vi "rs3 capture single 2.vi"(0 "queue in":u64, 5 "timeout":u32=5000, 11 "error in (no error)":errorcluster) -> (1 "Capture Error":string="No Error", 2 "Frame number":u64, 3 "RS Format":u16(ring)=6 items=["    RS2_FORMAT_ANY             , /**< When passed to enable stream, librealsense will try to provide best suited format */", "    RS2_FORMAT_Z16             , /**< 16-bit linear depth values. The depth is meters is equal to depth scale * pixel value. */", "    RS2_FORMAT_DISPARITY16     , /**< 16-bit linear disparity values. The depth in meters is equal to depth scale / pixel value. */", "    RS2_FORMAT_XYZ32F          , /**< 32-bit floating point 3D coordinates. */", "    RS2_FORMAT_YUYV            , /**< Standard YUV pixel format as described in https://en.wikipedia.org/wiki/YUV */", "    RS2_FORMAT_RGB8            , /**< 8-bit red, green and blue channels */", "    RS2_FORMAT_BGR8            , /**< 8-bit blue, green, and red channels -- suitable for OpenCV */", "    RS2_FORMAT_RGBA8           , /**< 8-bit red, green and blue channels + constant alpha channel equal to FF */", "    RS2_FORMAT_BGRA8           , /**< 8-bit blue, green, and red channels + constant alpha channel equal to FF */", "    RS2_FORMAT_Y8              , /**< 8-bit per-pixel grayscale image */", "    RS2_FORMAT_Y16             , /**< 16-bit per-pixel grayscale image */", "    RS2_FORMAT_RAW10           , /**< Four 10-bit luminance values encoded into a 5-byte macropixel */", "    RS2_FORMAT_RAW16           , /**< 16-bit raw image */", "    RS2_FORMAT_RAW8            , /**< 8-bit raw image */", "    RS2_FORMAT_UYVY            , /**< Similar to the standard YUYV pixel format, but packed in a different order */", "    RS2_FORMAT_MOTION_RAW      , /**< Raw data from the motion sensor */", "    RS2_FORMAT_MOTION_XYZ32F   , /**< Motion data packed as 3 32-bit float values, for X, Y, and Z axis */", "    RS2_FORMAT_GPIO_RAW        , /**< Raw data from the external sensors hooked to one of the GPIO's */", "    RS2_FORMAT_COUNT             /**< Number of enumeration values. Not a valid input: intended to be used in for-loops. */"], 4 "RS Stream":u16(ring) items=["    RS2_STREAM_ANY,", "    RS2_STREAM_DEPTH                            , /**< Native stream of depth data produced by RealSense device */", "    RS2_STREAM_COLOR                            , /**< Native stream of color data captured by RealSense device */", "    RS2_STREAM_INFRARED                         , /**< Native stream of infrared data captured by RealSense device */", "    RS2_STREAM_FISHEYE                          , /**< Native stream of fish-eye (wide) data captured from the dedicate motion camera */", "    RS2_STREAM_GYRO                             , /**< Native stream of gyroscope motion data produced by RealSense device */", "    RS2_STREAM_ACCEL                            , /**< Native stream of accelerometer motion data produced by RealSense device */", "    RS2_STREAM_GPIO                             , /**< Signals from external device connected through GPIO */", "    RS2_STREAM_COUNT"], 6 "frame out":u64, 8 "width":i32, 9 "Blocking time, ms":u32, 10 "Stream type":T1(ring), 12 "index":i32, 13 "Time stamp":dbl, 14 "height":i32, 15 "error out":errorcluster)   [LabVIEW 2018, in "libRealSense3.lvlib"]
doc: "This VI waits for and returns the FRAME handle of captured data. (This is a BLOCKING call)\nIt also queries the frame profile to identify the type of stream data it was. \nThis type is output into the \"Stream Type\":\n\n0 Depth\n3 Color left\n5 IR Left \n9 IR Right\n21 IR Left (Y16)\n25 IR RIght (Y16)"
uses:
  libRealSense3.lvlib
panel:
  # "RS3 Capture Single 2"
  # "(C) Intel Corp. 2017,  AGJ"
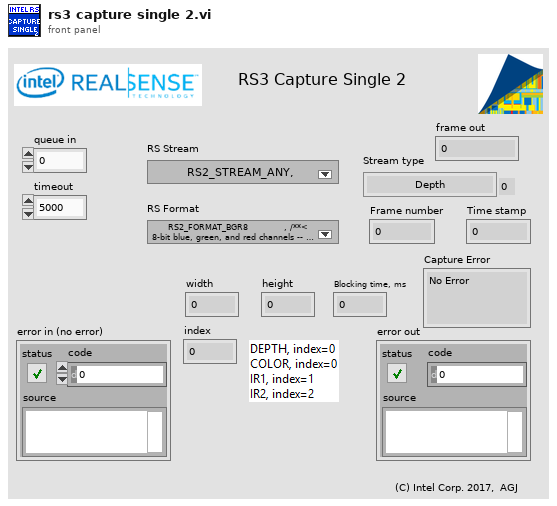
[diagram p1: front panel]
types:
  T1 = enum16{"Depth", "Color (ext.)", "Color (left) ", "IR Left", "IR Right", "IR Left (Y16)", "IR Right (Y16)"}
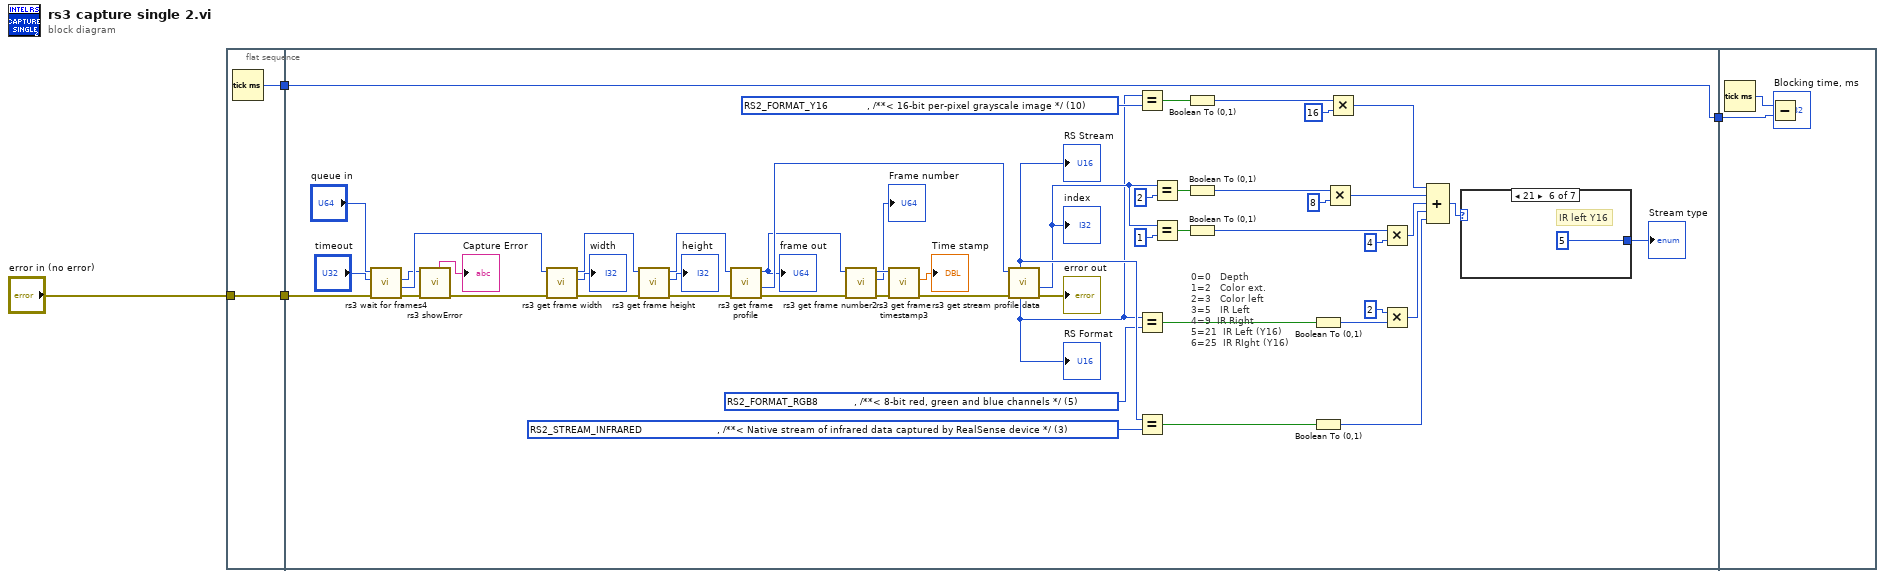
[diagram p0: block diagram]
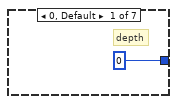
[diagram p2: hidden frame]
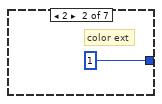
[diagram p3: hidden frame]
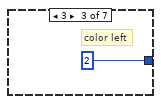
[diagram p4: hidden frame]
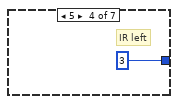
[diagram p5: hidden frame]
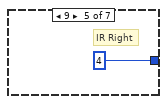
[diagram p6: hidden frame]
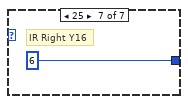
[diagram p7: hidden frame]
diagram:
  n1 = flat-sequence {
    tunnel: "error in (no error)" -> [w6]
    tunnel: [w6] -> w3
    tunnel: [w5] -> w2
    tunnel: w3 -> [w47]
    tunnel: w2 -> [w7]
    tunnel: [w7] -> w1
    tunnel: w1 -> [w67]
    frame #0 {
      n2 = Tick Count (ms)() -> (millisecond timer value=w5:u32)
    }
    frame #1 {
      w22 = u16 10 items=["    RS2_FORMAT_ANY             , /**< When passed to enable stream, librealsense will try to provide best suited format */", "    RS2_FORMAT_Z16             , /**< 16-bit linear depth values. The depth is meters is equal to depth scale * pixel value. */", "    RS2_FORMAT_DISPARITY16     , /**< 16-bit linear disparity values. The depth in meters is equal to depth scale / pixel value. */", "    RS2_FORMAT_XYZ32F          , /**< 32-bit floating point 3D coordinates. */", "    RS2_FORMAT_YUYV            , /**< Standard YUV pixel format as described in https://en.wikipedia.org/wiki/YUV */", "    RS2_FORMAT_RGB8            , /**< 8-bit red, green and blue channels */", "    RS2_FORMAT_BGR8            , /**< 8-bit blue, green, and red channels -- suitable for OpenCV */", "    RS2_FORMAT_RGBA8           , /**< 8-bit red, green and blue channels + constant alpha channel equal to FF */", "    RS2_FORMAT_BGRA8           , /**< 8-bit blue, green, and red channels + constant alpha channel equal to FF */", "    RS2_FORMAT_Y8              , /**< 8-bit per-pixel grayscale image */", "    RS2_FORMAT_Y16             , /**< 16-bit per-pixel grayscale image */", "    RS2_FORMAT_RAW10           , /**< Four 10-bit luminance values encoded into a 5-byte macropixel */", "    RS2_FORMAT_RAW16           , /**< 16-bit raw image */", "    RS2_FORMAT_RAW8            , /**< 8-bit raw image */", "    RS2_FORMAT_UYVY            , /**< Similar to the standard YUYV pixel format, but packed in a different order */", "    RS2_FORMAT_MOTION_RAW      , /**< Raw data from the motion sensor */", "    RS2_FORMAT_MOTION_XYZ32F   , /**< Motion data packed as 3 32-bit float values, for X, Y, and Z axis */", "    RS2_FORMAT_GPIO_RAW        , /**< Raw data from the external sensors hooked to one of the GPIO's */", "    RS2_FORMAT_COUNT             /**< Number of enumeration values. Not a valid input: intended to be used in for-loops. */"] ("RS Format")
      w44 = u16 3 items=["    RS2_STREAM_ANY,", "    RS2_STREAM_DEPTH                            , /**< Native stream of depth data produced by RealSense device */", "    RS2_STREAM_COLOR                            , /**< Native stream of color data captured by RealSense device */", "    RS2_STREAM_INFRARED                         , /**< Native stream of infrared data captured by RealSense device */", "    RS2_STREAM_FISHEYE                          , /**< Native stream of fish-eye (wide) data captured from the dedicate motion camera */", "    RS2_STREAM_GYRO                             , /**< Native stream of gyroscope motion data produced by RealSense device */", "    RS2_STREAM_ACCEL                            , /**< Native stream of accelerometer motion data produced by RealSense device */", "    RS2_STREAM_GPIO                             , /**< Signals from external device connected through GPIO */", "    RS2_STREAM_COUNT"] ("RS Stream")
      w21 = u16 5 items=["    RS2_FORMAT_ANY             , /**< When passed to enable stream, librealsense will try to provide best suited format */", "    RS2_FORMAT_Z16             , /**< 16-bit linear depth values. The depth is meters is equal to depth scale * pixel value. */", "    RS2_FORMAT_DISPARITY16     , /**< 16-bit linear disparity values. The depth in meters is equal to depth scale / pixel value. */", "    RS2_FORMAT_XYZ32F          , /**< 32-bit floating point 3D coordinates. */", "    RS2_FORMAT_YUYV            , /**< Standard YUV pixel format as described in https://en.wikipedia.org/wiki/YUV */", "    RS2_FORMAT_RGB8            , /**< 8-bit red, green and blue channels */", "    RS2_FORMAT_BGR8            , /**< 8-bit blue, green, and red channels -- suitable for OpenCV */", "    RS2_FORMAT_RGBA8           , /**< 8-bit red, green and blue channels + constant alpha channel equal to FF */", "    RS2_FORMAT_BGRA8           , /**< 8-bit blue, green, and red channels + constant alpha channel equal to FF */", "    RS2_FORMAT_Y8              , /**< 8-bit per-pixel grayscale image */", "    RS2_FORMAT_Y16             , /**< 16-bit per-pixel grayscale image */", "    RS2_FORMAT_RAW10           , /**< Four 10-bit luminance values encoded into a 5-byte macropixel */", "    RS2_FORMAT_RAW16           , /**< 16-bit raw image */", "    RS2_FORMAT_RAW8            , /**< 8-bit raw image */", "    RS2_FORMAT_UYVY            , /**< Similar to the standard YUYV pixel format, but packed in a different order */", "    RS2_FORMAT_MOTION_RAW      , /**< Raw data from the motion sensor */", "    RS2_FORMAT_MOTION_XYZ32F   , /**< Motion data packed as 3 32-bit float values, for X, Y, and Z axis */", "    RS2_FORMAT_GPIO_RAW        , /**< Raw data from the external sensors hooked to one of the GPIO's */", "    RS2_FORMAT_COUNT             /**< Number of enumeration values. Not a valid input: intended to be used in for-loops. */"] ("RS Format")
      # "0=0   Depth\n1=2   Color ext.\n2=3   Color left\n3=5   IR Left \n4=9  IR Right\n5=21  IR Left (Y16)\n6=25  IR RIght (Y16)"
      n3 = call "rs3 wait for frames4.vi"("error in (no error)"=w47, "timeout"="timeout", "Queue in"="queue in") -> (0:"error out"=w9:errorcluster, "frame"=w56:u64, 2:"error out"=w48:u64)  [unwired: 5 in, 1 out]
      n4 = call "rs3 showError.vi"("error in (no error)"=w9, "error"=w48) -> ("error out"=w8:errorcluster, "Error summary"=→"Capture Error":string)  [unwired: 5 in, 3 out]
      n5 = call "rs3 get frame width.vi"("error in (no error)"=w8, "frame in"=w56) -> ("error out"=w50:errorcluster, "width"=→"width":i32, "Frame out"=w54:u64)  [unwired: 6 in, 1 out]
      n6 = call "rs3 get frame height.vi"("error in (no error)"=w50, "frame in"=w54) -> ("error out"=w51:errorcluster, "height"=→"height":i32, "Frame out"=w55:u64)  [unwired: 6 in, 1 out]
      n7 = call "rs3 get frame profile.vi"("error in (no error)"=w51, "Frame"=w55) -> ("error out"=w14:errorcluster, "stream profile"=w49:u64, "frame out"=w18:u64)  [unwired: 6 in, 1 out]
      "frame out" <- w18
      n8 = call "rs3 get frame number2.vi"("error in (no error)"=w14, "frame in"=w18) -> ("error out"=w13:errorcluster, "Frame number"=→"Frame number":u64, "frame out"=w17:u64)  [unwired: 6 in, 1 out]
      n9 = call "rs3 get frame timestamp3.vi"("error in (no error)"=w13, "frame in"=w17) -> ("error out"=w12:errorcluster, "Time stamp"=→"Time stamp":dbl)  [unwired: 6 in, 2 out]
      n10 = call "rs3 get stream profile data.vi"("error in (no error)"=w12, "Profile"=w49) -> ("error out"=→"error out":errorcluster, "index"=w27:i32, "RS Format"=w19:u16, "RS Stream"=w43:u16)  [unwired: 2 in, 4 out]
      "RS Format" <- w19
      "RS Stream" <- w43
      "index" <- w27
      n11 = Equal?(x=w19, y=w22) -> (x = y?=w23:bool)
      n12 = Equal?(x=w19, y=w21) -> (x = y?=w40:bool)
      n13 = Equal?(x=w43, y=w44) -> (x = y?=w39:bool)
      n14 = Equal?(x=w27, y=2) -> (x = y?=w29:bool)
      n15 = Equal?(x=w27, y=1) -> (x = y?=w41:bool)
      n16 = Boolean To (0,1)(Boolean=w23) -> (0, 1=w25:i16)
      n17 = Boolean To (0,1)(Boolean=w29) -> (0, 1=w30:i16)
      n18 = Boolean To (0,1)(Boolean=w41) -> (0, 1=w36:i16)
      n19 = Boolean To (0,1)(Boolean=w40) -> (0, 1=w38:i16)
      n20 = Boolean To (0,1)(Boolean=w39) -> (0, 1=w33:i16)
      n21 = Multiply(x=w30, y=i16 8) -> (x*y=w26:i16)
      n22 = Multiply(x=w25, y=i16 16) -> (x*y=w20:i16)
      n23 = Multiply(x=w36, y=i16 4) -> (x*y=w32:i16)
      n24 = Multiply(x=i16 2, y=w38) -> (x*y=w34:i16)
      n25 = Compound Arithmetic op=ADD(w20, w26, w32, w34, w33) -> (w11:i16)
      n26 = case shown="21" w11 {
        tunnel: [0 1 2 3 4 5 6] -> w10
        frame 0, Default {
          # "depth"
        }
        frame 2 {
          # "color ext"
        }
        frame 3 {
          # "color left"
        }
        frame 5 {
          # "IR left"
        }
        frame 9 {
          # "IR Right"
        }
        frame 21 {
          # "IR left Y16"
        }
        frame 25 {
          # "IR Right Y16"
        }
      }
      "Stream type" <- w10
    }
    frame #2 {
      n27 = Tick Count (ms)() -> (millisecond timer value=w68:u32)
      n28 = Subtract(x=w68, y=w67) -> (x-y=→"Blocking time, ms":u32)
    }
  }
